vi "IniPotentiometer.vi"(9 "Invert Output":bool, 10 "refnum name":string="My Pot RefNum", 11 "Analog Channel":T1) -> ()   [LabVIEW 2018]
uses:
  <vilib>/Rock Robotics/SystemInterfaces/AI/FPGA_AIChannel.ctl
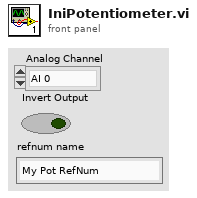
[diagram p1: front panel]
types:
  T1 = typedef "FPGA_AIChannel.ctl" = enum8{"AI 0", "AI 1", "AI 2", "AI 3", "AI MXP 0", "AI MXP 1", "AI MXP 2", "AI MXP 3", "Invalid"}
  T2 = typedef "WPI_PotentiometerDevRef.ctl" = cluster{"DevStatus":errorcluster, "Analog Channel":T1, "Invert Output":bool}
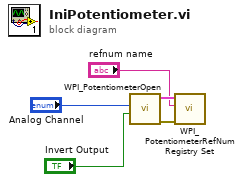
[diagram p0: block diagram]
diagram:
  n1 = call <vilib>:"WPI_PotentiometerOpen.vi"("Invert Output"="Invert Output", "Analog Channel"="Analog Channel") -> ("error out"=w5:errorcluster, "PotDevRef"=w4:T2)  [unwired: 8 in]
  n2 = call <vilib>:"WPI_PotentiometerRefNum Registry Set.vi"("error in (no error)"=w5, "refnum name"="refnum name", "PotDevRef"=w4) -> ()  [unwired: 7 in, 2 out]
